vi "setFrequencyViewer.vi"(8 "error in (no error)":errorcluster, 10 "Hardware:FrequencyCounters:FrequencyViewer.lvclass":refnum<class "FrequencyViewer.lvclass">, 11 "frequencyCounterController.lvclass in":refnum<class "frequencyCounterController.lvclass">) -> (0 "error out":errorcluster, 3 "frequencyCounterController.lvclass out":refnum<class "frequencyCounterController.lvclass">)   [LabVIEW 2009, in "Hardware.lvlib" / "frequencyCounters.lvlib" / "frequencyCounterController.lvclass"]
uses:
  frequencyCounterController.lvclass
  FrequencyViewer/FrequencyViewer.lvclass
  frequencyCounterController.lvclass/frequencyCounterController.ctl
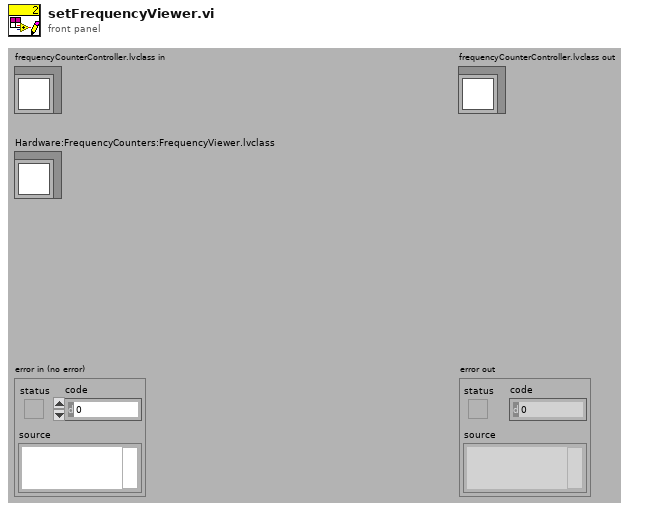
[diagram p1: front panel]
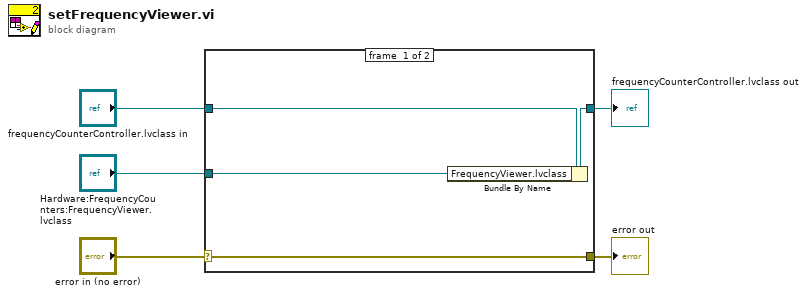
[diagram p0: block diagram]
diagram:
  n1 = case shown="No Error" "error in (no error)" {
    selector: "error in (no error)" -> [w9 w10]
    tunnel: [w9 w10] -> w4
    tunnel: [w7 w11] -> w2
    tunnel: "frequencyCounterController.lvclass in" -> [w8 w11]
    tunnel: "Hardware:FrequencyCounters:FrequencyViewer.lvclass" -> [w6 _]
    frame #0 {
      n2 = Bundle By Name(cluster=w8, "FrequencyViewer.lvclass"=w6) -> (w7:refnum<class "frequencyCounterController.lvclass">)
    }
    frame #1 {
    }
  }
  "error out" <- w4
  "frequencyCounterController.lvclass out" <- w2
